vi "Schedule Modify.vi"(9 "servings":i32, 10 "seconds":dbl, 11 "sched in":T1) -> (3 "sched out":T1)   [LabVIEW 2019, in "Pet Feeder.lvlib"]
uses:
  Pet Feeder.lvlib
  Controls/Feeder Program.ctl
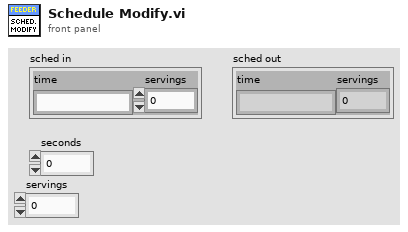
[diagram p1: front panel]
types:
  T1 = typedef "Pet Feeder.lvlib/Feeder Program.ctl" = cluster{"time":string, "servings":i32}
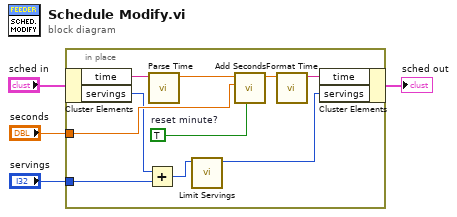
[diagram p0: block diagram]
diagram:
  n1 = in-place {
    in-place-border: "seconds" -> [w10]
    in-place-border: "servings" -> [w8]
    w5 = TRUE  # reset minute?
    n2 = in-place-cluster #1("sched in") -> ("time"=w14:string, "servings"=w9:i32)
    n3 = Add(x=w9, y=w8) -> (x+y=w7:i32)
    n4 = call "Parse Time.vi"("parse time"=w14) -> ("time (HH:MM:SS)"=w13:dbl)  [unwired: 10 in]
    n5 = call "Limit Servings.vi"("servings"=w7) -> ("coerced"=w6:i32)  [unwired: 10 in]
    n6 = call "Add Seconds.vi"("reset minute?"=w5, "seconds"=w10, "time in"=w13) -> ("time out"=w12:dbl)  [unwired: 8 in]
    n7 = call "Format Time.vi"("time (HH:MM:SS)"=w12) -> ("time string"=w11:string)  [unwired: 10 in]
    n8 = in-place-cluster #1("time"=w11, "servings"=w6) -> (→"sched out":T1)
  }
